vi "ShowHideInstructions.vi"(9 "Show/Hide":bool, 10 "Data Cluster":T1, 11 "VI in":refnum<vi>) -> ()   [LabVIEW 2020]
doc: "Shows or hides the picture with application instructions and adjusts front panel size and other controls."
uses:
  controls/UI Data.ctl
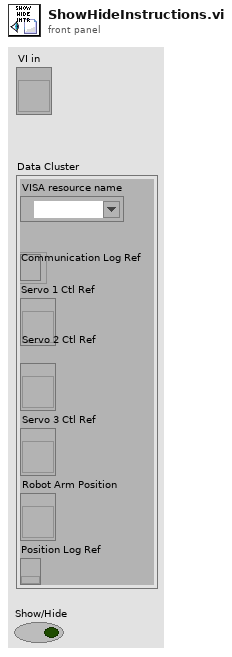
[diagram p1: front panel]
types:
  T1 = typedef "UI Data.ctl" = cluster{"VISA resource name":refnum<visa-resource-name>, "\nCommunication Log Ref":refnum<file>, "Servo 1 Ctl Ref":refnum<vi>, "Servo 2 Ctl Ref":refnum<vi>, "Servo 3 Ctl Ref":refnum<vi>, "Robot Arm Position":refnum<vi>, "Position Log Ref":refnum<k34>}
  T2 = typedef "LVRectTypeDef.ctl" = cluster{"Left":i16, "Top":i16, "Right":i16, "Bottom":i16}
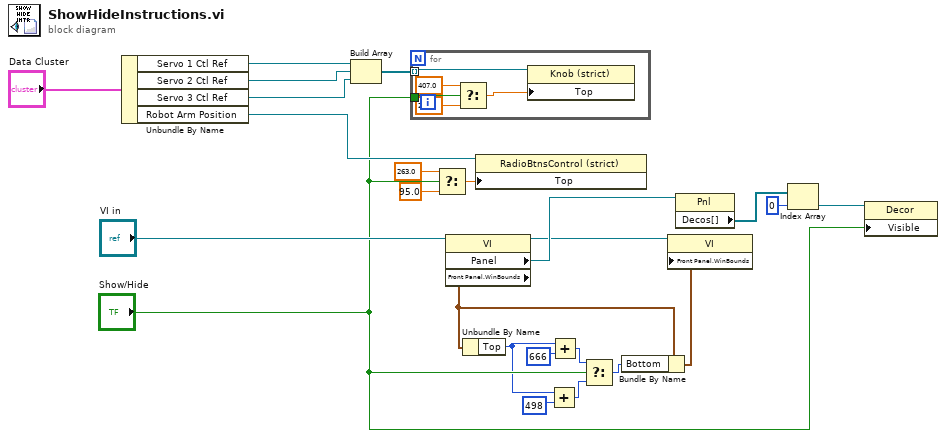
[diagram p0: block diagram]
diagram:
  n1 = Unbundle By Name("Data Cluster") -> ("Servo 1 Ctl Ref"=w16:refnum<vi>, "Servo 2 Ctl Ref"=w17:refnum<vi>, "Servo 3 Ctl Ref"=w18:refnum<vi>, "Robot Arm Position"=w20:refnum<vi>)
  n2 = Build Array(w16, w17, w18) -> (w19:refnum<vi>[])
  n3 = for {
    tunnel: w19 -> [w29] mode=indexing
    tunnel: "Show/Hide" -> [w28]
    n4 = Select(t=407.0, s=w28, f=239.0) -> (s? t:f=w27:dbl)
    n5 = property class="Knob (strict)"(reference=w29, "Top"=w27) -> ()  [unwired: 1 in, 2 out]
  }
  n6 = Select(t=263.0, s="Show/Hide", f=95.0) -> (s? t:f=w23:dbl)
  n7 = property class="VI"(reference="VI in") -> (reference out=w12:refnum<vi>, "Panel"=w13:refnum<vi>, "Front Panel.WinBounds"=w9:T2)  [unwired: 1 in, 1 out]
  n8 = Unbundle By Name(w9) -> ("Top"=w6:i16)
  n9 = property class="RadioBtnsControl (strict)"(reference=w20, "Top"=w23) -> ()  [unwired: 1 in, 2 out]
  n10 = Add(x=w6, y=i16 498) -> (x+y=w5:i16)
  n11 = Add(x=w6, y=i16 666) -> (x+y=w4:i16)
  n12 = Select(t=w4, s="Show/Hide", f=w5) -> (s? t:f=w11:i16)
  n13 = Bundle By Name(cluster=w9, "Bottom"=w11) -> (w10:T2)
  n14 = property class="VI"(reference=w12, "Front Panel.WinBounds"=w10) -> ()  [unwired: 1 in, 2 out]
  n15 = property class="Pnl"(reference=w13) -> ("Decos[]"=w1:refnum<vi>[])  [unwired: 1 in, 2 out]
  n16 = Index Array(array=w1, index=0) -> (element=w8:refnum<vi>)
  n17 = property class="Decor"(reference=w8, "Visible"="Show/Hide") -> ()  [unwired: 1 in, 2 out]
